vi "About Alligator.vi"() -> ()   [LabVIEW 2021, in "AlliGator GUI.lvlib"]
doc: "Modal \"About\" window for AlliGator."
uses:
  AlliGator GUI.lvlib
  Globals, Variables, Constants/AlliGator Globals.vi
  Globals, Variables, Constants/AlliGator Globals, Variables & Constants.lvlib
  Strings/Strings.lvlib
  Notebook/Notebook.lvlib
  Rich Text Box/Rich Text Box.lvlib
panel:
  out "Message":string
  in  "Beta":bool
  out "Version":string
  out "Alligator":string="  AlliGator"
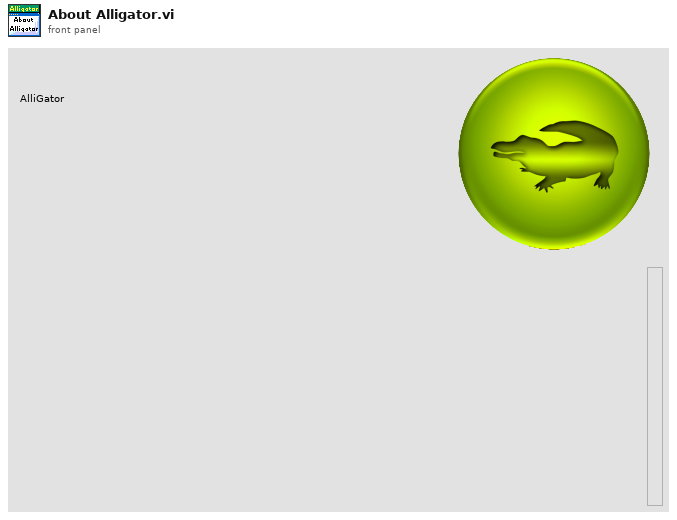
[diagram p1: front panel]
types:
  T1 = enum32{"Invalid", "Standard", "Closed", "Hidden", "Minimized", "Maximized"}
  T2 = typedef "Rich Text Box.lvlib/Text Formatting.ctl" = cluster{"Font":string, "Text Color":T3, "Text Background Color":T3, "Text Style":enum16{"Regular", "Bold", "Italic", "Underline", "Strikeout"}, "Font Size (Points)":dbl, "Text Alignment":i32}
  T3 = typedef "Rich Text Box.lvlib/Text Colors.ctl" = enum16{"Unchanged", "Black", "Blue", "Brown", "Gray", "Green", "Orange", "Pink", "Red", "White"}
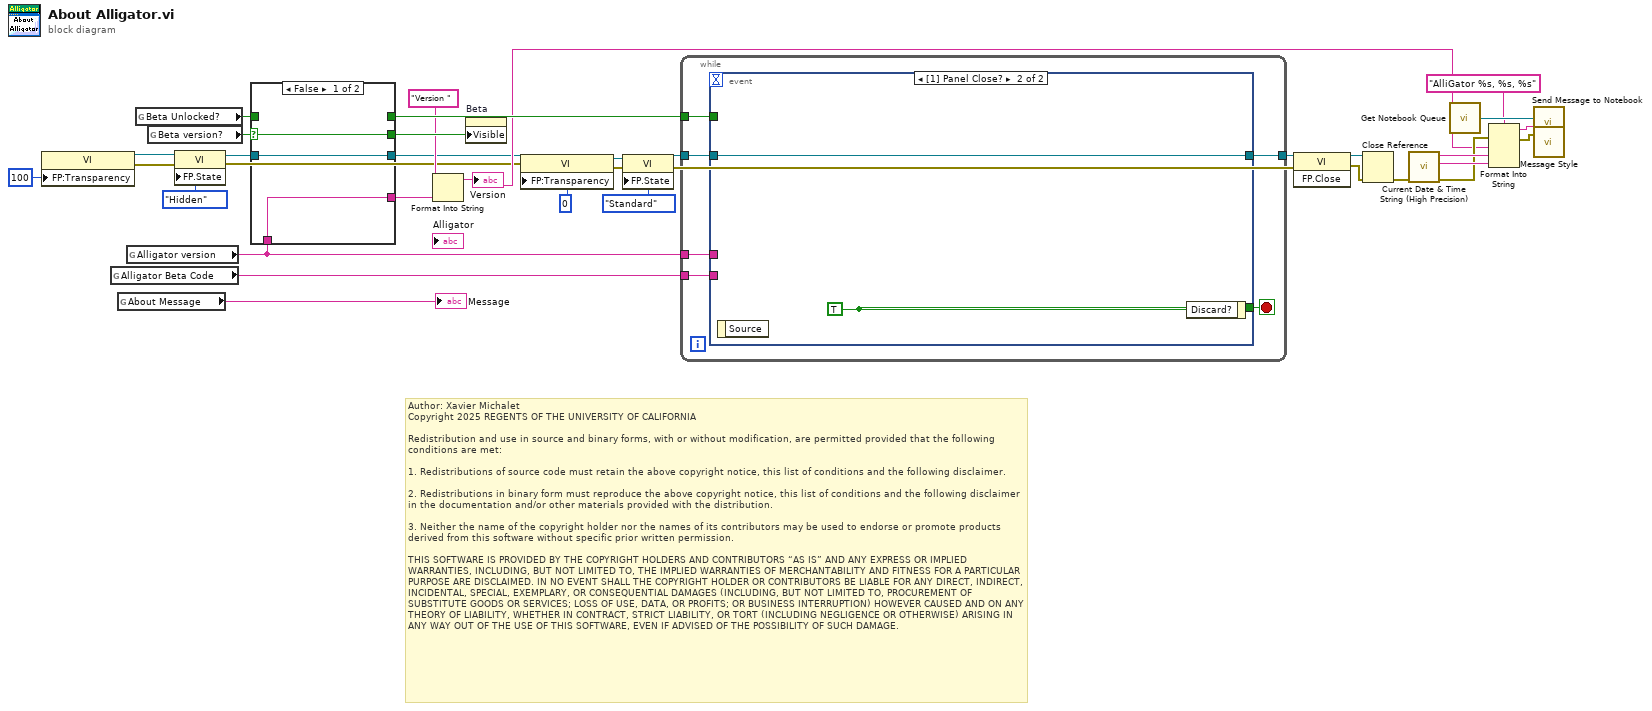
[diagram p0: block diagram]
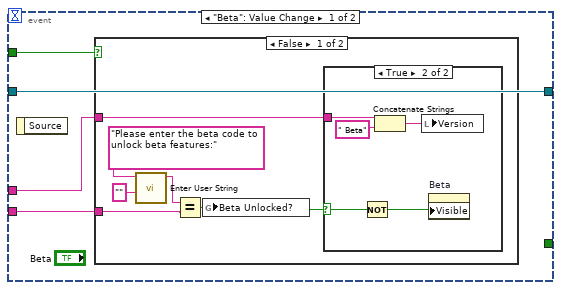
[diagram p2: hidden frame]
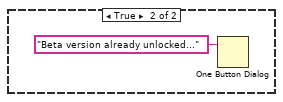
[diagram p4: hidden frame]
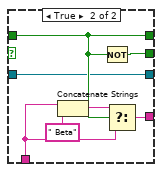
[diagram p5: hidden frame]
diagram:
  # "Author: Xavier Michalet\nCopyright 2025 REGENTS OF THE UNIVERSITY OF CALIFORNIA\n\nRedistribution and use in source and binary forms, with or without modification, are permitted provided that the following conditions are met:\n\n1. Redistributions of source code must retain the above copyright notice, this list of conditions and the following disclaimer.\n\n2. Redistributions in binary form must reproduce the above copyright notice, this list of conditions and the following disclaimer in the documentation and/or other materials provided with the distribution.\n\n3. Neither the name of the copyright holder nor the names of its contributors may be used to endorse or promote products derived from this software without specific prior written permission.\n\nTHIS SOFTWARE IS PROVIDED BY THE COPYRIGHT HOLDERS AND CONTRIBUTORS “AS IS” AND ANY EXPRESS OR IMPLIED WARRANTIES, INCLUDING, BUT NOT LIMITED TO, THE IMPLIED WARRANTIES OF MERCHANTABILITY AND FITNESS FOR A PARTICULAR PURPOSE ARE DISCLAIMED. IN NO EVENT SHALL THE COPYRIGHT HOLDER OR CONTRIBUTORS BE LIABLE FOR ANY DIRECT, INDIRECT, INCIDENTAL, SPECIAL, EXEMPLARY, OR CONSEQUENTIAL DAMAGES (INCLUDING, BUT NOT LIMITED TO, PROCUREMENT OF SUBSTITUTE GOODS OR SERVICES; LOSS OF USE, DATA, OR PROFITS; OR BUSINESS INTERRUPTION) HOWEVER CAUSED AND ON ANY THEORY OF LIABILITY, WHETHER IN CONTRACT, STRICT LIABILITY, OR TORT (INCLUDING NEGLIGENCE OR OTHERWISE) ARISING IN ANY WAY OUT OF THE USE OF THIS SOFTWARE, EVEN IF ADVISED OF THE POSSIBILITY OF SUCH DAMAGE."
  n1 = property class="VI"("FP:Transparency"=u8 100 ("Front Panel Window:Transparency")) -> (reference out=w11:refnum<vi>, error out=w10:errorcluster)  [unwired: 2 in]
  n2 = global read "AlliGator Globals.vi" "Alligator Beta Code"() -> (w32:string)
  n3 = global read "AlliGator Globals.vi" "About Message"() -> (→"Message":string)
  n4 = global read "AlliGator Globals.vi" "Alligator version"() -> (w29:string)
  n5 = global read "AlliGator Globals.vi" "Beta Unlocked?"() -> (w17:bool)
  n6 = global read "AlliGator Globals.vi" "Beta version?"() -> (w28:bool)
  n7 = property class="VI"(reference=w11, error in=w10, "FP.State"=T1."Hidden" ("Front Panel Window:State")) -> (reference out=w9:refnum<vi>, error out=w4:errorcluster)
  n8 = case shown="False" w28 {
    selector: w28 -> [w37 _]
    tunnel: [w36 w43] -> w15
    tunnel: [w37 w42] -> w31
    tunnel: [_ w39] -> w30
    tunnel: w29 -> [w36 w40]
    tunnel: w17 -> [_ w39]
    tunnel: w9 -> [w35 w38]
    tunnel: [w35 w38] -> w7
    frame False {
    }
    frame True {
      n9 = Concatenate Strings(w40, " Beta" ("string")) -> (w41:string)
      n10 = Not(x=w39) -> (.not. x?=w42:bool)
      n11 = Select(t=w41, s=w39, f=w40) -> (s? t:f=w43:string)
    }
  }
  n12 = Format Into String(initial string="Version ", w15) -> (resulting string=w16:string)  [unwired: 2 in, 1 out]
  "Version" <- w16
  n13 = property on="Beta" class="Bool"("Visible"=w31) -> ()  [unwired: 2 in, 2 out]
  n14 = property class="VI"(reference=w7, error in=w4, "FP:Transparency"=u8 0 ("Front Panel Window:Transparency")) -> (reference out=w6:refnum<vi>, error out=w5:errorcluster)
  n15 = property class="VI"(reference=w6, error in=w5, "FP.State"=T1."Standard" ("Front Panel Window:State")) -> (error out=w2:errorcluster)  [unwired: 1 out]
  n16 = while {
    tunnel: [w48] -> w34
    tunnel: w6 -> [w49]
    tunnel: w29 -> [w47]
    tunnel: w30 -> [w46]
    tunnel: w32 -> [w45]
    stop <- w50 stop-if-true
    n17 = event shown="[1] Panel Close?" {
      selector: _ -> [_ _]
      dyn-events: _ -> [_ _]
      timeout: _ -> [_ _]
      tunnel: [_ w68] -> w50
      tunnel: w49 -> [w51 w67]
      tunnel: [w51 w67] -> w48
      tunnel: w47 -> [w52 _]
      tunnel: w46 -> [w54 _]
      tunnel: w45 -> [w53 _]
      event "Beta": Value Change {
        n18 = event-data() -> ()  [unwired: 1 in, 1 out]
        n19 = case shown="False" w54 {
          tunnel: w53 -> [w60 _]
          tunnel: w52 -> [w57 _]
          frame False {
            n20 = call "Enter User String.vi"("Caption"="", "Message"="Please enter the beta code to unlock beta features:") -> ("User entered string"=w59:string)  [unwired: 7 in, 2 out]
            n21 = Equal?(x=w59, y=w60) -> (x = y?=w58:bool)
            n22 = global write "AlliGator Globals.vi" "Beta Unlocked?"(w58) -> ()
            n23 = case shown="True" w58 {
              selector: w58 -> [_ w62]
              tunnel: w57 -> [_ w65]
              frame False {
              }
              frame True {
                n24 = Not(x=w62) -> (.not. x?=w61:bool)
                n25 = Concatenate Strings(w65, " Beta" ("string")) -> (w63:string)
                n26 = local write "Version"(w63) -> ()
                n27 = property on="Beta" class="Bool"("Visible"=w61) -> ()  [unwired: 2 in, 2 out]
              }
            }
          }
          frame True {
            n28 = One Button Dialog(message="Beta version already unlocked...") -> ()  [unwired: 1 in, 1 out]
          }
        }
      }
      event Panel Close? {
        w68 = TRUE ("Discard?")
        n29 = event-data() -> ()  [unwired: 1 in, 1 out]
        n30 = event-data("Discard?"=w68) -> ()  [unwired: 1 in, 1 out]
      }
    }
  }
  n31 = invoke class="VI" method="FP.Close"(reference=w34, error in=w2) -> (reference out=w33:refnum<vi>, error out=w18:errorcluster)  [unwired: 1 in, 1 out]
  n32 = Close Reference(reference=w33, error in (no error)=w18) -> (error out=w19:errorcluster)
  n33 = call "Current Date & Time String (High Precision).vi"("Error In"=w19) -> ("Error Out"=w25:errorcluster, "time string"=w27:string, "date string"=w26:string)  [unwired: 7 in, 1 out]
  n34 = call "Get Notebook Queue.vi"() -> ("Notebook Queue"=w21:refnum<queue>)  [unwired: 9 in]
  n35 = Format Into String(format string="AlliGator %s, %s, %s" ("initial string"), error in=w25, w16, w26, w27) -> (resulting string=w23:string, error out=w24:errorcluster)  [unwired: 1 in]
  n36 = call "Message Style.vi"() -> ("Message Formatting"=w22:T2)
  n37 = call "Send Message to Notebook.vi"("Text Formatting"=w22, "Error In"=w24, "Message"=w23, "Notebook Queue"=w21) -> ()  [unwired: 4 in, 2 out]
